vi "5492_TalonVelocityToRPM.vi"(11 "Talon Velocity":dbl) -> (3 "RPM":dbl)   [LabVIEW 2016]
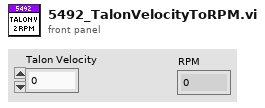
[diagram p1: front panel]
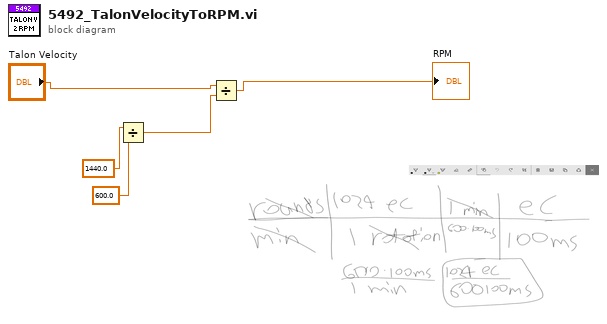
[diagram p0: block diagram]
diagram:
  n1 = Divide(x=1440.0, y=600.0) -> (x/y=w3:dbl)
  n2 = Divide(x="Talon Velocity", y=w3) -> (x/y=→"RPM":dbl)
